vi "Actor Core.vi"(8 "error in (no error)":errorcluster, 11 "Test Actors in":refnum<class "Test Actors.lvclass">) -> (0 "error out":errorcluster, 3 "Actor out":refnum<class "Actor.lvclass">)   [LabVIEW 2015, in "Test Actors.lvclass"]
uses:
  Test Actors.lvclass
  <vilib>/ActorFramework/Actor/Actor.lvclass
  Test Interface/Test Interface.lvclass
  Mag Lab Measure Base/Mag Lab Measure Base.lvclass/Mag Lab Measure Base.ctl
  Mag Lab Root/Mag Lab Root.lvclass/Mag Lab Root.ctl
  <vilib>/ActorFramework/Actor/Actor.lvclass/Actor.ctl
  <vilib>/ActorFramework/Message Enqueuer/Message Enqueuer.lvclass/Message Enqueuer.ctl
  Mag Lab Root/Write Separate UI.vi
  <vilib>/ActorFramework/Message Enqueuer/Init from Existing Queue.vi
  <vilib>/ActorFramework/Message Enqueuer/Enqueue.vi
  <vilib>/ActorFramework/Message Priority Queue/Priority Enqueue.vi
  Mag Lab Measure Base/Mag Lab Measure Base.lvclass
  <vilib>/ActorFramework/Message Enqueuer/Message Enqueuer.lvclass
  Mag Lab Measure Base Messages/Launch Inteface Msg/Launch Inteface Msg.lvclass
panel:
  # "Test core"
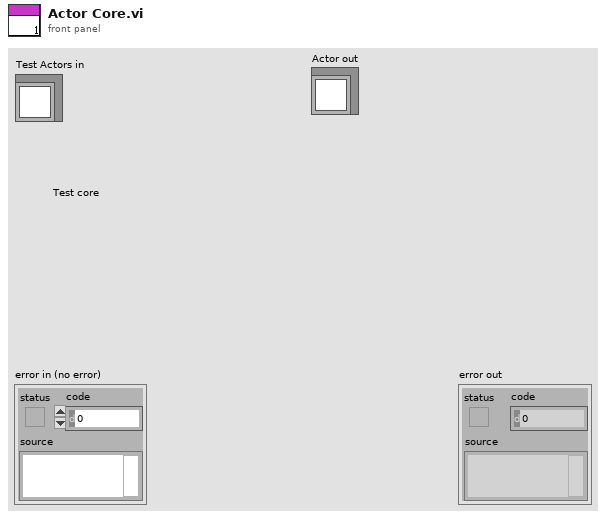
[diagram p1: front panel]
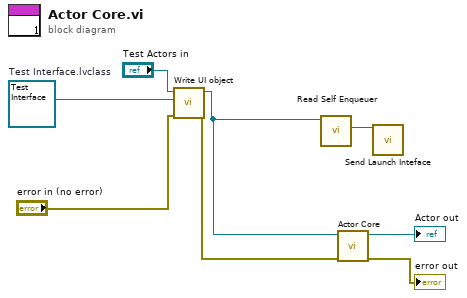
[diagram p0: block diagram]
diagram:
  w3 = refnum<class "Test Interface.lvclass"> refnum  # Test Interface.lvclass
  n1 = call "Write UI object.vi"("error in (no error)"="error in (no error)", "Mag Lab Measure Interface.lvclass"=w3, "Mag Lab Measure Base in"="Test Actors in") -> ("error out"=w1:errorcluster, "Mag Lab Measure Base out"=w4:refnum<class "Test Actors.lvclass">)  [unwired: 7 in]
  n2 = call <vilib>:"Read Self Enqueuer.vi"("Actor"=w4) -> ("Self Enqueuer"=w6:refnum<class "Message Enqueuer.lvclass">)  [unwired: 10 in]
  n3 = call-parent "Actor Core.vi"("error in"=w1, "Mag Lab Measure Base in"=w4) -> ("error out"=→"error out":errorcluster, "Actor out"=→"Actor out":refnum<class "Actor.lvclass">)  [unwired: 8 in]
  n4 = call "Send Launch Inteface.vi"("Message Enqueuer"=w6) -> ()  [unwired: 9 in, 2 out]
